vi "DDPoseEst2_Rel_TrajCreation.vi"(9 "Effective Track Width Ft":dbl=5.83 format="%17.3f", 11 "Max Velocity Ft/Sec":dbl=5.55 format="%17.3f") -> (0 "Trajectory  creation error":errorcluster, 1 "Relative Trajectory":T2 {"States"."POSE"."ROTATION"."SIN" format="%13.4f"; "States"."POSE"."ROTATION"."COS" format="%13.4f"; "States"."POSE"."ROTATION"."VALUE" format="%13.4f"; "States"."POSE"."TRANSLATION"."Y" format="%14.3f"; "States"."POSE"."TRANSLATION"."X" format="%14.3f"; "TotalTImeSecs" format="%20.3f"}, 2 "Trajectory Items":i32, 3 "TotalTImeSecs":dbl)   [LabVIEW 2019]
uses:
  <vilib>/Rock Robotics/WPI/ThirdParty/JAS_Junk/TrajLib/TypeDef/DISPLAY_WEIGHTED_WAYPOINT.ctl
  <vilib>/Rock Robotics/WPI/ThirdParty/JAS_Junk/TrajLib/Enum/TRAJECTORY_SPLINE_TYPE_ENUM.ctl
  <vilib>/Rock Robotics/WPI/ThirdParty/JAS_Junk/TrajLib/TypeDef/TRAJECTORY.ctl
  <vilib>/Rock Robotics/WPI/ThirdParty/JAS_Junk/TrajLib/TypeDef/TRAJ_STATE.ctl
  <vilib>/Rock Robotics/WPI/ThirdParty/JAS_Junk/TrajLib/TypeDef/POSE2D.ctl
  <vilib>/Rock Robotics/WPI/ThirdParty/JAS_Junk/TrajLib/TypeDef/TRANSLATION2D.ctl
  <vilib>/Rock Robotics/WPI/ThirdParty/JAS_Junk/TrajLib/TypeDef/ROTATION2D.ctl
  <vilib>/Rock Robotics/WPI/ThirdParty/JAS_Junk/TrajLib/Conv_Deg_Radians.vi
  <vilib>/Rock Robotics/WPI/ThirdParty/JAS_Junk/TrajLib/Util_DispWeightedWaypoint_To_WeightedWayPoint.vi
  <vilib>/Rock Robotics/SystemInterfaces/NetworkCommunication/NetComm_UsageReport_report.vi
  <vilib>/Rock Robotics/WPI/ThirdParty/JAS_Junk/TrajLib/DiffDriveKinematicsConstraint_New.vi
  <vilib>/Rock Robotics/WPI/ThirdParty/JAS_Junk/TrajLib/TrajectoryConfig_AddConstraint.vi
  <vilib>/Rock Robotics/WPI/ThirdParty/JAS_Junk/TrajLib/CentripetalAccelConstraint_New.vi
  <vilib>/Rock Robotics/WPI/ThirdParty/JAS_Junk/TrajLib/Translation2d_Create.vi
  <vilib>/Rock Robotics/WPI/ThirdParty/JAS_Junk/TrajLib/Rotation2d_CreateAngle.vi
  <vilib>/Rock Robotics/WPI/ThirdParty/JAS_Junk/TrajLib/Globals/Util_LibraryGlobals.vi
  <vilib>/Rock Robotics/WPI/ThirdParty/JAS_Junk/TrajLib/Trajectory_Library.lvlib
panel:
  in  "Interior Waypoint 2":T1={"X"=210.0, "Y"=106.0, "ANGLE"=45.0, "WEIGHT"=2.0} {"WEIGHT" format="%13.3f"; "ANGLE" format="%13.3f"; "Y" format="%13.3f"; "X" format="%13.3f"}
  out "Trajectory":cluster{dbl[], dbl[]}[](graph)
  in  "Spline Type":T7
  in  "Interior Waypoint 1":T1={"X"=105.0, "Y"=65.0, "ANGLE"=0.0, "WEIGHT"=2.0} {"WEIGHT" format="%13.3f"; "ANGLE" format="%13.3f"; "Y" format="%13.3f"; "X" format="%13.3f"}
  in  "Destination Waypoint":T1={"X"=300.0, "Y"=65.0, "ANGLE"=-45.0, "WEIGHT"=2.0} {"WEIGHT" format="%13.3f"; "ANGLE" format="%13.3f"; "Y" format="%13.3f"; "X" format="%13.3f"}
  in  "Initial Waypoint":T1={"X"=15.0, "Y"=105.0, "ANGLE"=-45.0, "WEIGHT"=2.0} {"WEIGHT" format="%13.3f"; "ANGLE" format="%13.3f"; "Y" format="%13.3f"; "X" format="%13.3f"}
  in  "Use Diff Drive\nKinematic\nConstraint":bool=TRUE
  in  "Use Centripetal\nAcceleration\nConstaint":bool=TRUE
  out "Track Width_M":dbl=0.66 format="%20.4f"
  out "MaxAcceleration  M/S^2":dbl=1.3 format="%17.4f"
  out "MaxVelocity M/S":dbl=2.0 format="%17.4f"
  out "Max Cent Accel":dbl=1.0 format="%20.4f"
  in  "Max Cent Accel INCHES/SEC^2":dbl=15.0 format="%20.1f"
  in  "MaxAcceleration INCHES/SEC^2":dbl=30.0 format="%17.1f"
  in  "MaxVelocity Fraction":dbl=0.66 format="%17.3f"
  # "This VI is designed to be called by BEGIN.VI, but can be executed directly to test trajectory parameters."
  # "CREATED TRAJECTORY INFORMATION"
  # "TRAJECTORY CONFIGURATION"
  # "real sim robot 20.9 inch"
  # "TRAJECTORY DEFINITION"
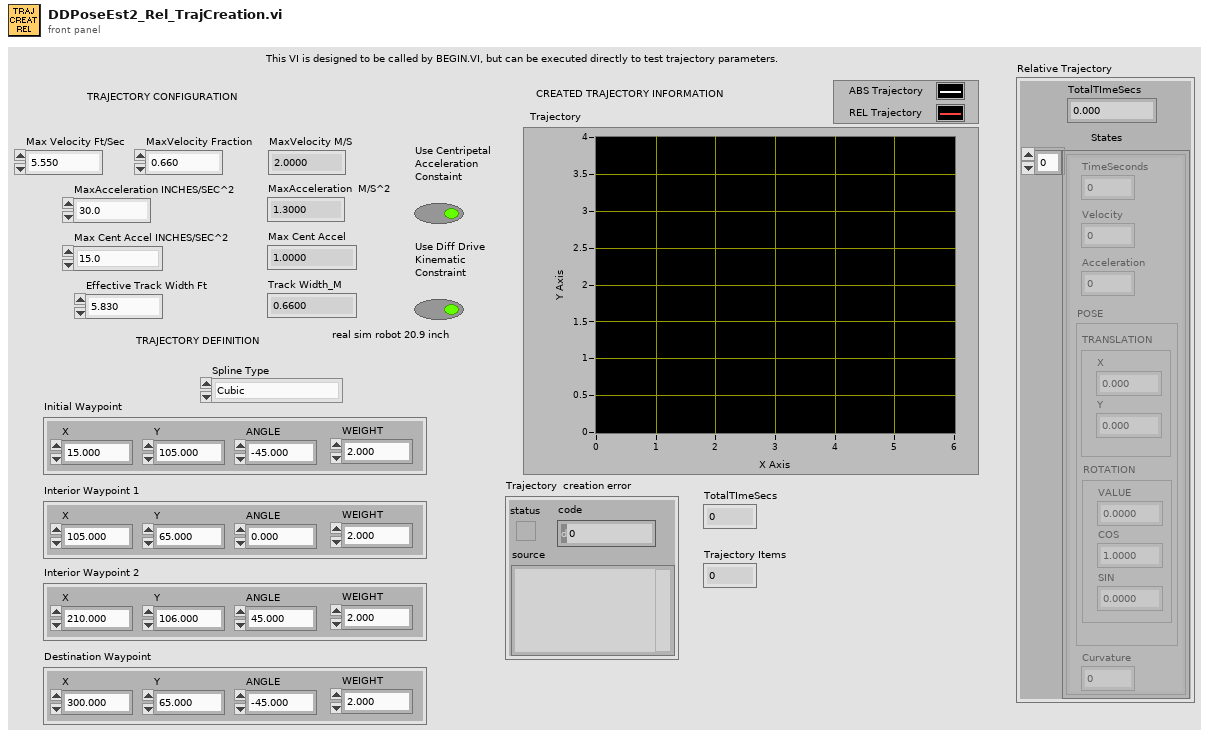
[diagram p1: front panel]
types:
  T1 = typedef "Trajectory_Library.lvlib/DISPLAY_WEIGHTED_WAYPOINT.ctl" = cluster{"X":dbl, "Y":dbl, "ANGLE":dbl, "WEIGHT":dbl}
  T2 = typedef "Trajectory_Library.lvlib/TRAJECTORY.ctl" = cluster{"TotalTImeSecs":dbl, "States":T3[]}
  T3 = typedef "Trajectory_Library.lvlib/TRAJ_STATE.ctl" = cluster{"TimeSeconds":dbl, "Velocity":dbl, "Acceleration":dbl, "POSE":T4, "Curvature":dbl}
  T4 = typedef "Trajectory_Library.lvlib/POSE2D.ctl" = cluster{"TRANSLATION":T5, "ROTATION":T6}
  T5 = typedef "Trajectory_Library.lvlib/TRANSLATION2D.ctl" = cluster{"X":dbl, "Y":dbl}
  T6 = typedef "Trajectory_Library.lvlib/ROTATION2D.ctl" = cluster{"VALUE":dbl, "COS":dbl, "SIN":dbl}
  T7 = typedef "Trajectory_Library.lvlib/TRAJECTORY_SPLINE_TYPE_ENUM.ctl" = enum16{"Cubic", "Cubic With Weights", "Quintic", "Quintic With Weights"}
  T8 = typedef "Trajectory_Library.lvlib/WEIGHTED_WAYPOINT.ctl" = cluster{"TRANSLATION":T5, "ROTATION":T6, "SCALAR":dbl}
  T9 = typedef "Trajectory_Library.lvlib/TRAJ_CONFIG.ctl" = cluster{"MaxVelocity":dbl, "Max Acceleration":dbl, "StartVelocity":dbl, "End Velocity":dbl, "Reversed":bool, "Constraints":variant[]}
  T10 = typedef "Trajectory_Library.lvlib/DIFF_DRIVE_KINEMATICS.ctl" = cluster{"TrackWidth_Meters":dbl}
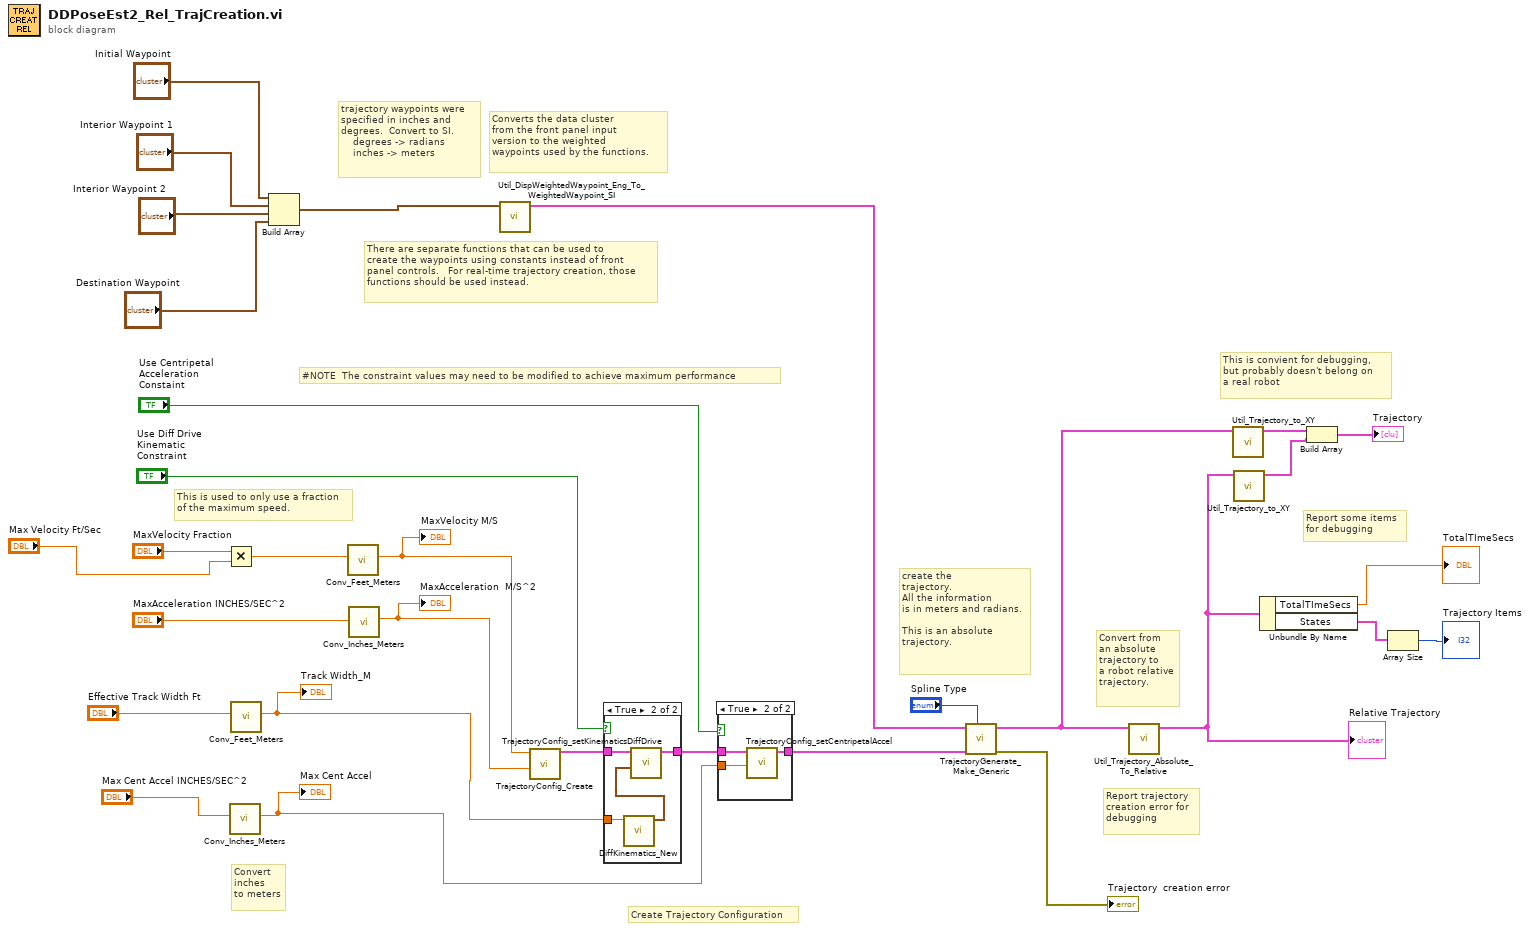
[diagram p0: block diagram]
diagram:
  # "There are separate functions that can be used to \ncreate the waypoints using constants instead of front\npanel controls.   For real-time trajectory creation, those\nfunctions should be used instead."
  # "This is convient for debugging,\nbut probably doesn't belong on\na real robot"
  # "This is used to only use a fraction\nof the maximum speed."
  # "Report trajectory\ncreation error for \ndebugging"
  # "Report some items\nfor debugging"
  # "Converts the data cluster\nfrom the front panel input\nversion to the weighted \nwaypoints used by the functions."
  # "#NOTE  The constraint values may need to be modified to achieve maximum performance"
  # "Convert from\nan absolute\ntrajectory to\na robot relative\ntrajectory."
  # "Convert\ninches\nto meters"
  # "create the\ntrajectory.\nAll the information\nis in meters and radians.\n\nThis is an absolute \ntrajectory."
  # "trajectory waypoints were \nspecified in inches and\ndegrees.  Convert to SI.\n    degrees -> radians\n    inches -> meters"
  # "Create Trajectory Configuration"
  n1 = Multiply(x="MaxVelocity Fraction", y="Max Velocity Ft/Sec") -> (x*y=w16:dbl)
  n2 = call <vilib>:"Conv_Inches_Meters.vi"("INCH"="Max Cent Accel INCHES/SEC^2") -> ("Meters"=w24:dbl)  [unwired: 10 in]
  "Max Cent Accel" <- w24
  n3 = call <vilib>:"Conv_Feet_Meters.vi"("Feet"="Effective Track Width Ft") -> ("Meters"=w25:dbl)  [unwired: 10 in]
  "Track Width_M" <- w25
  n4 = Build Array("Initial Waypoint", "Interior Waypoint 1", "Interior Waypoint 2", "Destination Waypoint") -> (w11:T1[])
  n5 = call <vilib>:"Conv_Feet_Meters.vi"("Feet"=w16) -> ("Meters"=w22:dbl)  [unwired: 10 in]
  "MaxVelocity M/S" <- w22
  n6 = call <vilib>:"Conv_Inches_Meters.vi"("INCH"="MaxAcceleration INCHES/SEC^2") -> ("Meters"=w23:dbl)  [unwired: 10 in]
  "MaxAcceleration  M/S^2" <- w23
  n7 = call <vilib>:"Util_DispWeightedWaypoint_Eng_To_WeightedWaypoint_SI.vi"("DisplayWeightedWayPoints_ENG"=w11) -> ("WeightedWayPoints_SI"=w10:T8[])  [unwired: 10 in]
  n8 = call <vilib>:"TrajectoryConfig_Create.vi"("MaxAcceleration"=w23, "MaxVelocity"=w22) -> ("TRAJECTORY_CONFIG"=w29:T9)  [unwired: 9 in]
  n9 = case shown="True" "Use Diff Drive\nKinematic\nConstraint" {
    tunnel: w29 -> [w32 w36]
    tunnel: [w32 w35] -> w28
    tunnel: w25 -> [_ w33]
    frame False {
    }
    frame True {
      n10 = call <vilib>:"DiffKinematics_New.vi"("TrackWidth_Meters"=w33) -> ("DIFF_DRIVE_KINEMATICS"=w34:T10)  [unwired: 10 in]
      n11 = call <vilib>:"TrajectoryConfig_setKinematicsDiffDrive.vi"("DIFF_DRIVE_KINEMATICS"=w34, "inTRAJECTORY_CONFIG"=w36) -> ("outTRAJECTORY_CONFIG"=w35:T9)  [unwired: 9 in]
    }
  }
  n12 = case shown="True" "Use Centripetal\nAcceleration\nConstaint" {
    tunnel: w28 -> [w37 w40]
    tunnel: [w37 w39] -> w20
    tunnel: w24 -> [_ w38]
    frame False {
    }
    frame True {
      n13 = call <vilib>:"TrajectoryConfig_setCentripetalAccel.vi"("Max Cent Accel"=w38, "inTRAJECTORY_CONFIG"=w40) -> ("outTRAJECTORY_CONFIG"=w39:T9)  [unwired: 9 in]
    }
  }
  n14 = call <vilib>:"TrajectoryGenerate_Make_Generic.vi"("Spline Type"="Spline Type", "traj_config"=w20, "WeightedWayPoints"=w10) -> ("error out"=→"Trajectory  creation error":errorcluster, "TRAJECTORY"=w9:T2)  [unwired: 7 in]
  n15 = call <vilib>:"Util_Trajectory_Absolute_To_Relative.vi"("absTRAJECTORY"=w9) -> ("outputRelativeTRAJECTORY"=w8:T2)  [unwired: 10 in]
  "Relative Trajectory" <- w8
  n16 = call <vilib>:"Util_Trajectory_to_XY.vi"("TRAJECTORY"=w9) -> ("outArrayXY"=w7:cluster{dbl[], dbl[]})  [unwired: 10 in]
  n17 = call <vilib>:"Util_Trajectory_to_XY.vi"("TRAJECTORY"=w8) -> ("outArrayXY"=w6:cluster{dbl[], dbl[]})  [unwired: 10 in]
  n18 = Unbundle By Name(w8) -> ("TotalTImeSecs"=→"TotalTImeSecs":dbl, "States"=w18:T3[])
  n19 = Build Array(w7, w6) -> (→"Trajectory":cluster{dbl[], dbl[]}[])
  n20 = Array Size(array=w18) -> (size(s)=→"Trajectory Items":i32)
